vi "Constructor by Info Cluster FK Ring.vi"(8 "error in (no error)":errorcluster, 9 "FK Ring Field Info":T1, 10 "Database (use member data)":refnum<class "Database.lvclass">, 11 "Field in":refnum<class "Field.lvclass">) -> (0 "error out":errorcluster, 3 "Field out":refnum<class "Field.lvclass">)   [LabVIEW 2020, in "Field.lvclass"]
uses:
  Field.lvclass
  Database.lvclass
  FK Ring Field Info.ctl
  FK Ring Info.ctl
  FK Ring.lvclass
  C:/Users/User/Desktop/Raman Program/Database OOP/source/Field/Field.lvclass
  Field.lvclass/Field.ctl
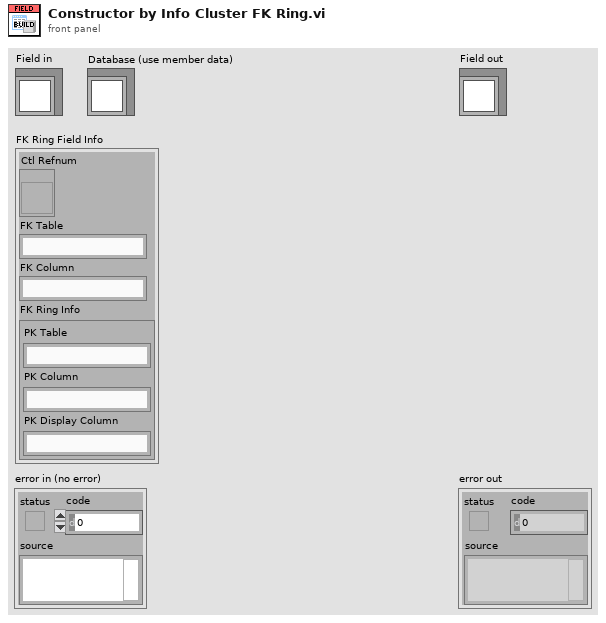
[diagram p1: front panel]
types:
  T1 = typedef "FK Ring Field Info.ctl" = cluster{"Ctl Refnum":refnum<vi>, "FK Table":string, "FK Column":string, "FK Ring Info":T2}
  T2 = typedef "FK Ring Info.ctl" = cluster{"PK Table":string, "PK Column":string, "PK Display Column":string}
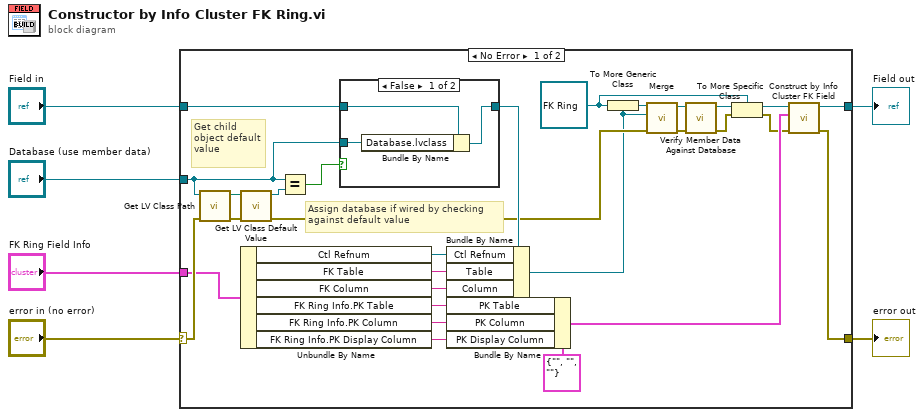
[diagram p0: block diagram]
diagram:
  n1 = case shown="No Error" "error in (no error)" {
    selector: "error in (no error)" -> [w29 w41]
    tunnel: [w24 w41] -> w5
    tunnel: [w25 w40] -> w3
    tunnel: "Field in" -> [w30 w40]
    tunnel: "Database (use member data)" -> [w31 _]
    tunnel: "FK Ring Field Info" -> [w21 _]
    frame No Error {
      w15 = refnum<class "FK Ring.lvclass"> refnum ("FK Ring.lvclass")
      # "Get child object default value"
      # "Assign database if wired by checking\nagainst default value"
      n2 = call <vilib>:"Get LV Class Path.vi"("error in (no error)"=w29, "object"=w31) -> ("error out"=w34:errorcluster, "class path"=w35:path)  [unwired: 8 in]
      n3 = call <vilib>:"Get LV Class Default Value.vi"("error in (no error)"=w34, "class path"=w35) -> ("error out"=w27:errorcluster, "object"=w33:refnum<class>)  [unwired: 8 in]
      n4 = Unbundle By Name(w21) -> ("Ctl Refnum"=w26:refnum<vi>, "FK Table"=w8:string, "FK Column"=w7:string, "FK Ring Info.PK Table"=w20:string, "FK Ring Info.PK Column"=w19:string, "FK Ring Info.PK Display Column"=w18:string)
      n5 = Equal?(x=w31, y=w33) -> (x = y?=w32:bool)
      n6 = case shown="False" w32 {
        tunnel: w31 -> [w37 _]
        tunnel: w30 -> [w38 w39]
        tunnel: [w36 w39] -> w28
        frame False {
          n7 = Bundle By Name(cluster=w38, "Database.lvclass"=w37) -> (w36:refnum<class "Field.lvclass">)
        }
        frame True {
        }
      }
      n8 = Bundle By Name(cluster=w28, "Ctl Refnum"=w26, "Table"=w8, "Column"=w7) -> (w17:refnum<class "Field.lvclass">)
      n9 = Bundle By Name(cluster=T2 {"PK Table"="", "PK Column"="", "PK Display Column"=""} ("FK Ring Info"), "PK Table"=w20, "PK Column"=w19, "PK Display Column"=w18) -> (w22:T2)
      n10 = To More Generic Class(target class=w17, reference=w15) -> (generic class reference=w16:refnum<class "Field.lvclass">)
      n11 = call-dynamic "Merge.vi"("error in (no error)"=w27, "Field To Merge"=w17, "Field In"=w16) -> ("error out"=w11:errorcluster, "Merged Field out"=w12:refnum<class "Field.lvclass">)  [unwired: 7 in]
      n12 = call-dynamic "Verify Member Data Against Database.vi"("error in (no error)"=w11, "Field in"=w12) -> ("error out"=w9:errorcluster, "Field out"=w10:refnum<class "Field.lvclass">)  [unwired: 8 in]
      n13 = To More Specific Class(target class=w15, reference=w10, error in=w9) -> (specific class reference=w14:refnum<class "FK Ring.lvclass">, error out=w13:errorcluster)
      n14 = call "Construct by Info Cluster FK Field.vi"("error in (no error)"=w13, "FK Ring Info"=w22, "FK Ring in"=w14) -> ("error out"=w24:errorcluster, "FK Ring out"=w25:refnum<class "FK Ring.lvclass">)  [unwired: 7 in]
    }
    frame Error {
    }
  }
  "error out" <- w5
  "Field out" <- w3
